vi "Write Numeric A.vi"(8 "error in (no error)":errorcluster, 10 "Double Float.lvclass":T1, 11 "Add in":refnum<class "AbsFunc_One Term_Complex DBL.lvclass">) -> (0 "error out":errorcluster, 3 "Add out":refnum<class "AbsFunc_One Term_Complex DBL.lvclass">)   [LabVIEW 2021, in "AbsFunc_One Term_Complex DBL.lvclass"]
uses:
  AbsFunc_One Term_Complex DBL.lvclass
  Support/Abstract Type.ctl
  Abs_Types/Complex Double Float/Abs_Complex Double Float.lvclass
  AbsFunc_One Term_Complex DBL.lvclass/AbsFunc_One Term_Complex DBL.ctl
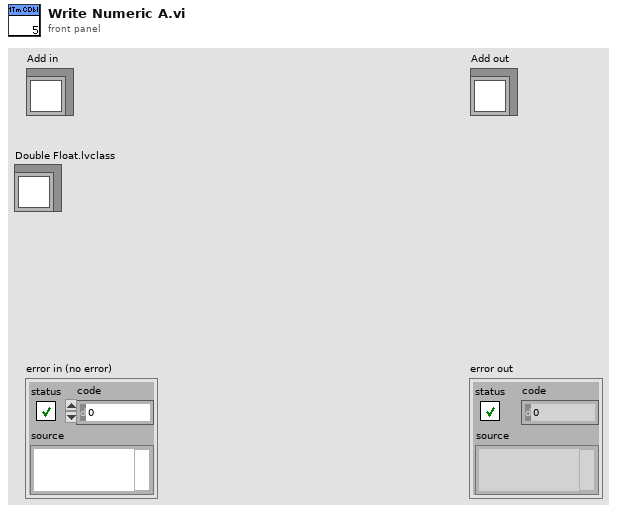
[diagram p1: front panel]
types:
  T1 = typedef "AbsFunc_One Term_Complex DBL.lvclass/Abstract Type.ctl" = refnum<class "Abs_Complex Double Float.lvclass">
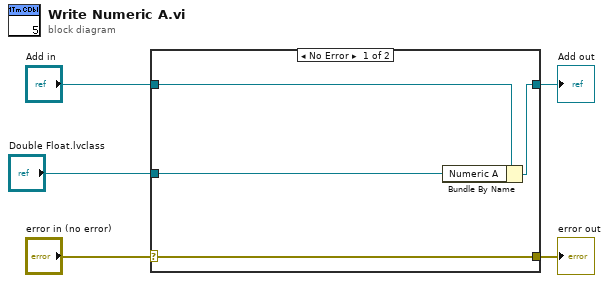
[diagram p0: block diagram]
diagram:
  n1 = case shown="No Error" "error in (no error)" {
    selector: "error in (no error)" -> [w9 w10]
    tunnel: [w9 w10] -> w4
    tunnel: [w7 w11] -> w2
    tunnel: "Add in" -> [w8 w11]
    tunnel: "Double Float.lvclass" -> [w6 _]
    frame No Error {
      n2 = Bundle By Name(cluster=w8, "Numeric A"=w6) -> (w7:refnum<class "AbsFunc_One Term_Complex DBL.lvclass">)
    }
    frame Error {
    }
  }
  "error out" <- w4
  "Add out" <- w2
